vi "T7 Stream Enable KAG.vi"(0 "IP:Port":string, 5 "Enable":enum32{"Disable", "Enable"}(ring), 11 "error in":errorcluster) -> (15 "error out":errorcluster)   [LabVIEW 2022 SP3]
doc: "Write Stream ENABLE LabJack Register via MODBUS."
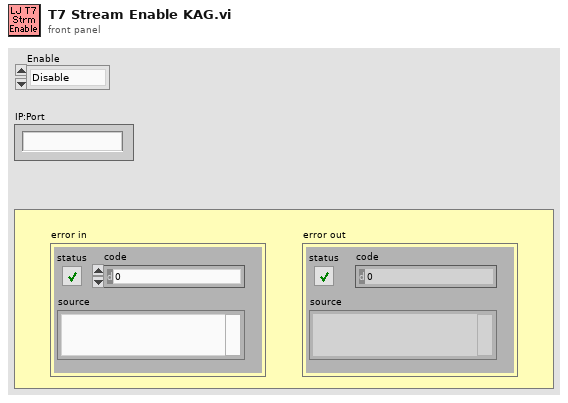
[diagram p1: front panel]
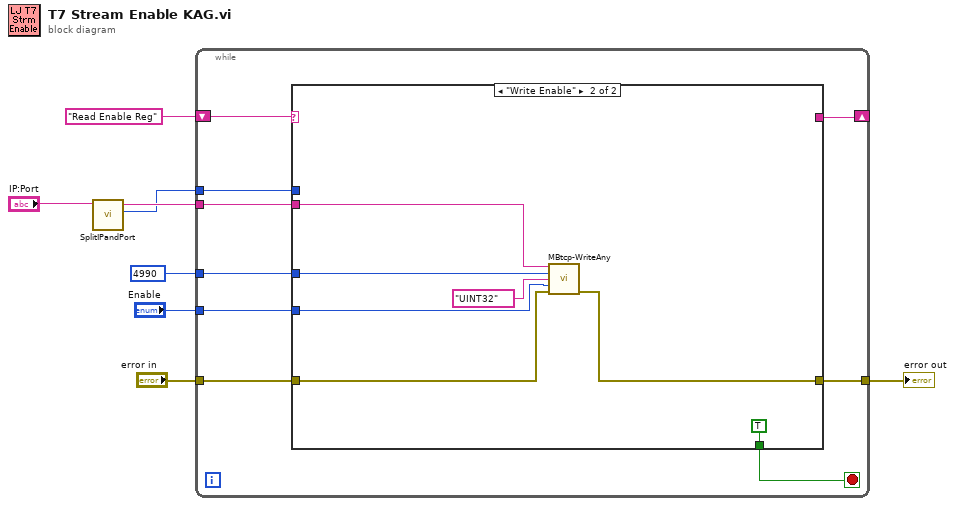
[diagram p0: block diagram]
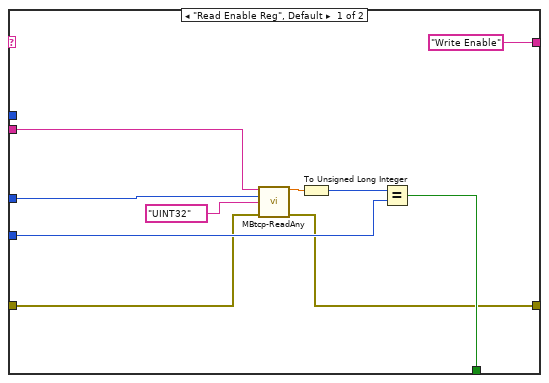
[diagram p2: hidden frame]
diagram:
  n1 = call "SplitIPandPort.vi"("IP:Port"="IP:Port") -> ("Port"=w2:u16, "IP"=w3:string)  [unwired: 9 in]
  n2 = while {
    shift-right: [w16] -> _
    shift-left: "Read Enable Reg" -> [w17]
    tunnel: "error in" -> [w15]
    tunnel: [w14] -> w6
    tunnel: w3 -> [w13]
    tunnel: "Enable" -> [w12]
    tunnel: 4990 ("LabJack UINT32 Register") -> [w11]
    tunnel: w2 -> [w9]
    stop <- w10 stop-if-true
    n3 = case shown="\"Write Enable\"" w17 {
      tunnel: ["Write Enable" _] -> w16
      tunnel: w15 -> [w23 w33]
      tunnel: [w18 w30] -> w14
      tunnel: w13 -> [w22 w31]
      tunnel: w12 -> [w26 w28]
      tunnel: w11 -> [w21 w32]
      tunnel: [w25 TRUE] -> w10
      tunnel: w9 -> [_ _]
      frame "Read Enable Reg", Default {
        n4 = call "MBtcp-ReadAny.vi"("IP Address"=w22, "Register"=w21, "DataType(:RegisterType)"="UINT32" ("Data type"), "Error In"=w23) -> ("Value"=w20:dbl, "error out"=w18:errorcluster)  [unwired: 9 in, 1 out]
        n5 = To Unsigned Long Integer(number=w20) -> (unsigned 32bit integer=w19:u32)
        n6 = Equal?(x=w19, y=w26) -> (x = y?=w25:bool)
      }
      frame "Write Enable" {
        n7 = call "MBtcp-WriteAny.vi"("IP Address"=w31, "Register"=w32, "DataType(:RegisterType)"="UINT32" ("Data type"), "Value to Output"=w28, "Error In"=w33) -> ("error out"=w30:errorcluster)  [unwired: 10 in]
      }
    }
  }
  "error out" <- w6
